vi "non_FPGA_VI.vi"() -> ()   [LabVIEW 2020]
uses:
  c5c29772-c0b0-45e0-ac49-cc5077cfdad3.vi
  <vilib>/Array/Sort 2D Array - Pop Stack.vi
  <vilib>/Array/Sort 2D Array - Push Stack.vi
  c5c29772-c0b0-45e0-ac49-cc5077cfdad3.vi/269d4b3b-47f5-49e3-8884-44851e4dd9d5.vi
  c5c29772-c0b0-45e0-ac49-cc5077cfdad3.vi/6d99389c-673d-4efb-bf33-19b32bcf4cf8.vi
  <vilib>/Analysis/NI_AALBase.lvlib
panel:
  out "sorted 2D array":dbl[][](array[numeric])
  out "appended array":dbl[][](array[numeric])
  out "Array 3":i32[](array[numeric])
  out "sorted array":dbl[](array[numeric])
  out "Array":dbl[](array[numeric])
  out "uniform white noise":dbl[](array[numeric])
  out "Waveform Graph":dbl[](graph)
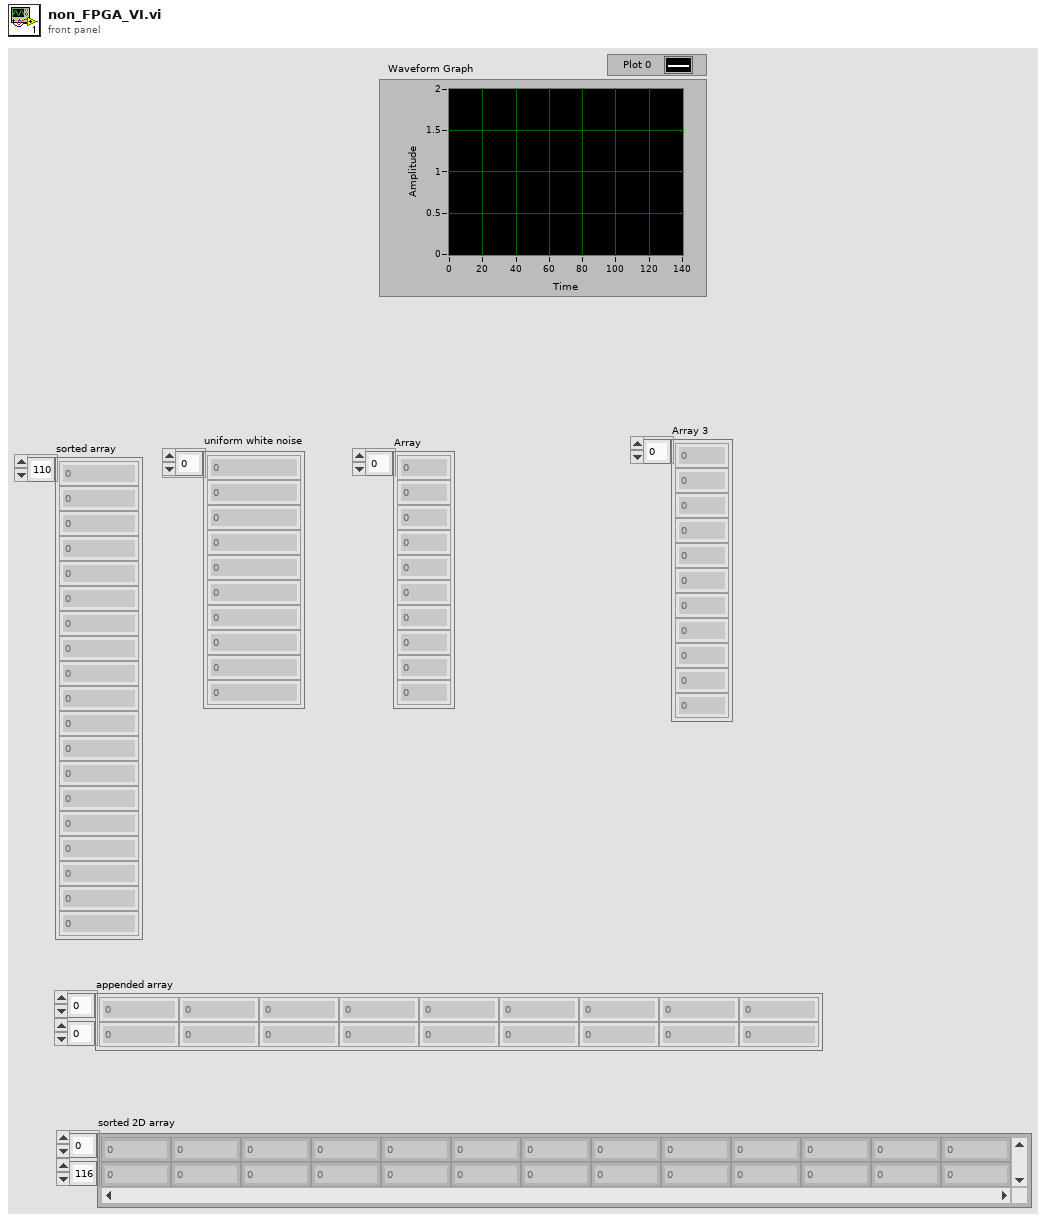
[diagram p1: front panel]
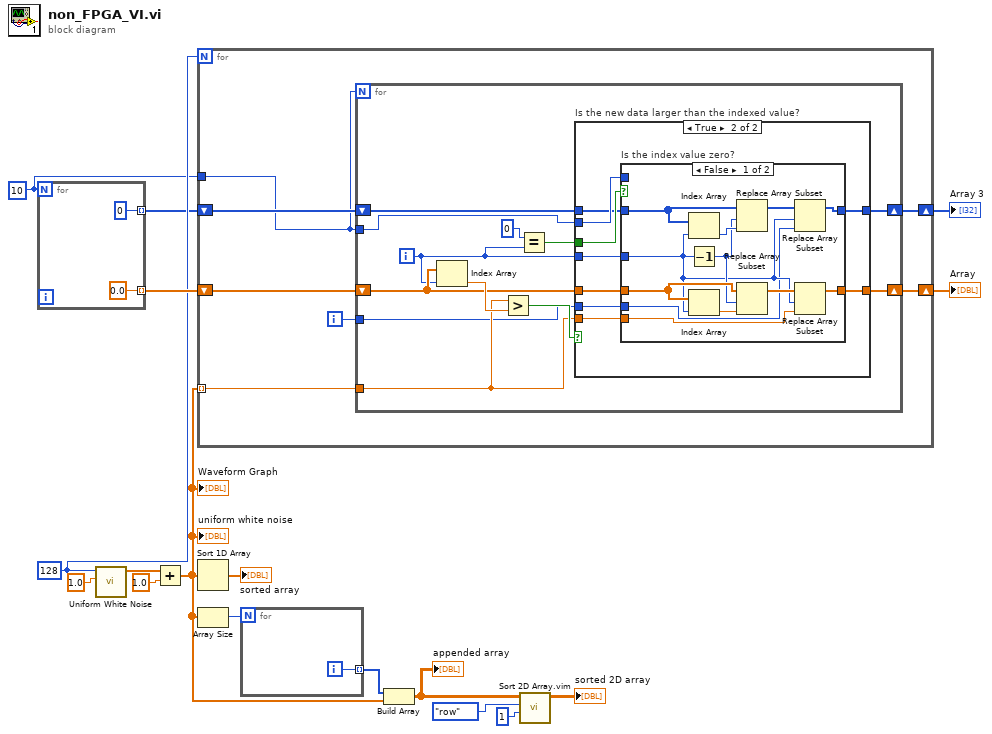
[diagram p0: block diagram]
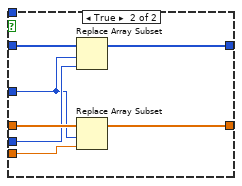
[diagram p3: hidden frame]
diagram:
  w1 = 10
  w13 = 128 ("samples")
  n1 = for {
    N: w1 -> [_]
    tunnel: [0.0 ("amplitude")] -> w16 mode=indexing
    tunnel: [0] -> w10 mode=indexing
  }
  n2 = call <vilib>:"Uniform White Noise.vi"("amplitude"=1.0, "samples"=w13) -> ("uniform white noise"=w8:dbl[])  [unwired: 8 in, 1 out]
  n3 = Add(x=w8, y=1.0 ("amplitude")) -> (x+y=w2:dbl[])
  "Waveform Graph" <- w2
  "uniform white noise" <- w2
  n4 = for {
    N: w13 -> [_]
    tunnel: w2 -> [w26] mode=indexing
    shift-right: [w24] -> w15
    shift-left: w16 -> [w25]
    shift-right: [w22] -> w11
    shift-left: w10 -> [w21]
    tunnel: w1 -> [w20]
    i -> [w23]
    n5 = for {
      N: w20 -> [_]
      tunnel: w26 -> [w33]
      tunnel: w20 -> [w31]
      shift-right: [w32] -> w24
      shift-left: w25 -> [w36]
      tunnel: w23 -> [w29]
      shift-right: [w27] -> w22
      shift-left: w21 -> [w28]
      i -> [w30]
      n6 = Index Array(array=w36, index=w30) -> (element=w38:dbl)
      n7 = Greater?(x=w33, y=w38) -> (0:w37:bool)
      n8 = Equal?(x=0, y=w30) -> (x = y?=w34:bool)
      n9 = case "Is the new data larger than the indexed value?" shown="True" w37 {
        tunnel: w36 -> [w40 w48]
        tunnel: w34 -> [_ w49]
        tunnel: w31 -> [_ w47]
        tunnel: w33 -> [_ w46]
        tunnel: w30 -> [_ w45]
        tunnel: [w40 w44] -> w32
        tunnel: w29 -> [_ w43]
        tunnel: w28 -> [w39 w42]
        tunnel: [w39 w41] -> w27
        frame False {
        }
        frame True {
          n10 = case "Is the index value zero?" shown="False" w49 {
            tunnel: w48 -> [w61 w68]
            tunnel: w47 -> [_ _]
            tunnel: w46 -> [w58 w67]
            tunnel: w45 -> [w51 w64]
            tunnel: [w57 w66] -> w44
            tunnel: w43 -> [w50 w65]
            tunnel: w42 -> [w54 w63]
            tunnel: [w53 w62] -> w41
            frame False {
              n11 = Index Array(array=w54, index=w51) -> (element=w56:i32)
              n12 = Decrement(x=w51) -> (x-1=w52:i32)
              n13 = Index Array(array=w61, index=w51) -> (element=w60:dbl)
              n14 = Replace Array Subset(array=w54, new element=w56, index=w52) -> (w55:i32[])
              n15 = Replace Array Subset(array=w61, new element=w60, index=w52) -> (w59:dbl[])
              n16 = Replace Array Subset(array=w55, new element=w50, index=w51) -> (w53:i32[])
              n17 = Replace Array Subset(array=w59, new element=w58, index=w51) -> (w57:dbl[])
            }
            frame True {
              n18 = Replace Array Subset(array=w63, new element=w65, index=w64) -> (w62:i32[])
              n19 = Replace Array Subset(array=w68, new element=w67, index=w64) -> (w66:dbl[])
            }
          }
        }
      }
    }
  }
  "Array" <- w15
  "Array 3" <- w11
  n20 = Sort 1D Array(array=w2) -> (sorted array=→"sorted array":dbl[])
  n21 = Array Size(array=w2) -> (size(s)=w9:i32)
  n22 = for {
    N: w9 -> [_]
    tunnel: [w69] -> w7 mode=indexing
    i -> [w69]
  }
  n23 = Build Array(w7, w2) -> (w6:dbl[][])
  "appended array" <- w6
  n24 = call "Sort 2D Array.vim"("index"=1, "dimension to index (column)"=enum16{"column", "row"}."row", "2D array"=w6) -> ("sorted 2D array"=→"sorted 2D array":dbl[][])  [unwired: 7 in, 1 out]
